vi "SetParent.vi"(8 "error in (no error)":errorcluster, 10 "hWndNewParent":i32, 11 "hWndChild":i32) -> (0 "error out":errorcluster, 3 "hWnd":i32)   [LabVIEW 2025, in "Test Unit.lvlib"]
uses:
  Test Unit.lvlib
  user32.dll
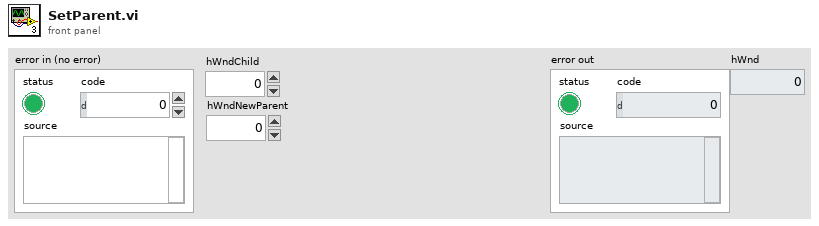
[diagram p1: front panel]
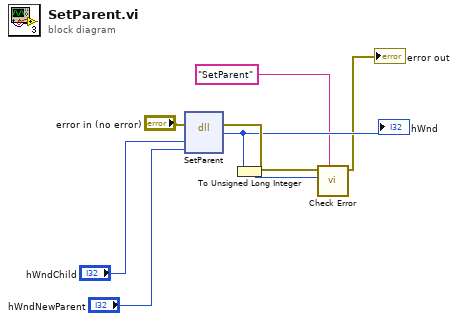
[diagram p0: block diagram]
diagram:
  n1 = dll-call lib="user32.dll" fn="SetParent"(error in="error in (no error)", "hWndChild"="hWndChild", "hWndNewParent"="hWndNewParent") -> (error out=w5:errorcluster, "hWnd"=w4:i32)  [unwired: 4 in, 1 out]
  "hWnd" <- w4
  n2 = To Unsigned Long Integer(number=w4) -> (unsigned 32bit integer=w1:u32)
  n3 = call "Check Error.vi"("Description"="SetParent", "Return Code"=w1, "error in (no error)"=w5) -> ("error out"=→"error out":errorcluster)  [unwired: 8 in]
